vi "Enable Concurrent Frequency.vi"(7 "Enable Concurrent Frequency(T: Enable)":bool=TRUE, 8 "error in (no error)":errorcluster, 10 "Channel (1: Channel 1)":u16(ring)=1 items=["Channel 1"=1, "Channel2"=2], 11 "VISA resource name":refnum<visa-resource-name>) -> (0 "error out":errorcluster, 3 "VISA resource name out":refnum<visa-resource-name>)   [LabVIEW 2016, in "Tektronix AFG 1000 Series.lvlib"]
doc: "Enables or disables the concurrent frequency of two channels. The frequency of the specified channel will be copied to the other channel. When the concurrent copy function is enabled, the FreqLock function is also enabled automaticlly."
uses:
  Tektronix AFG 1000 Series.lvlib
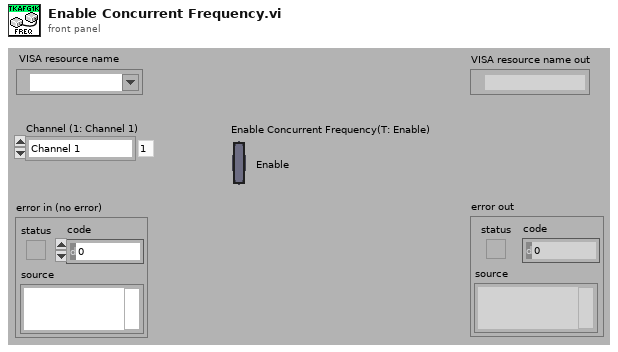
[diagram p1: front panel]
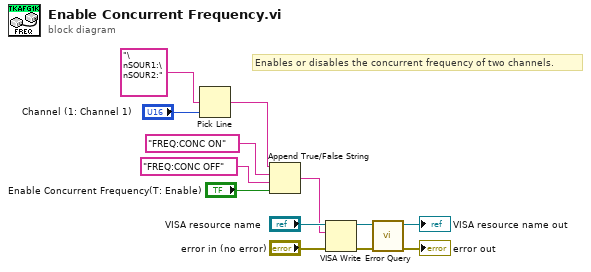
[diagram p0: block diagram]
diagram:
  # "Enables or disables the concurrent frequency of two channels."
  n1 = Pick Line(multi-line string="\nSOUR1:\nSOUR2:" ("string (\"\")"), line index="Channel (1: Channel 1)") -> (output string=w1:string)  [unwired: 1 in]
  n2 = Append True/False String(1:"Enable Concurrent Frequency(T: Enable)", 2:"FREQ:CONC OFF" ("true string"), 3:"FREQ:CONC ON" ("true string"), 4:w1) -> (0:w8:string)
  n3 = VISA Write(VISA resource name="VISA resource name", write buffer=w8, error in (no error)="error in (no error)") -> (VISA resource name out=w6:refnum<visa-resource-name>, error out=w7:errorcluster)  [unwired: 1 out]
  n4 = call "Error Query.vi"("error in (no error)"=w7, "VISA resource name"=w6) -> ("error out"=→"error out":errorcluster, "VISA resource name out"=→"VISA resource name out":refnum<visa-resource-name>)  [unwired: 6 in, 2 out]
